vi "licenses.vi"   [LabVIEW 2019]
uses:
  <vilib>/xml/Load XML File.vi
  <vilib>/xml/Close Reference(Node).vi
  <vilib>/Utility/config.llb/Read Key (String).vi
  <vilib>/xml/NI_XML.lvlib
  <vilib>/Utility/config.llb/NI_LVConfig.lvlib
panel:
  # "This VI reads the package information from the .vipc file,\nloads the license information from the VIPM package cache,\nand stores the license text into the licenses/ directory.\n\nImportant note: This VI will only work on Windows!"
types:
  T1 = typedef "NI_LVConfig.lvlib/Config Data RefNum.ctl" = refnum<k1>
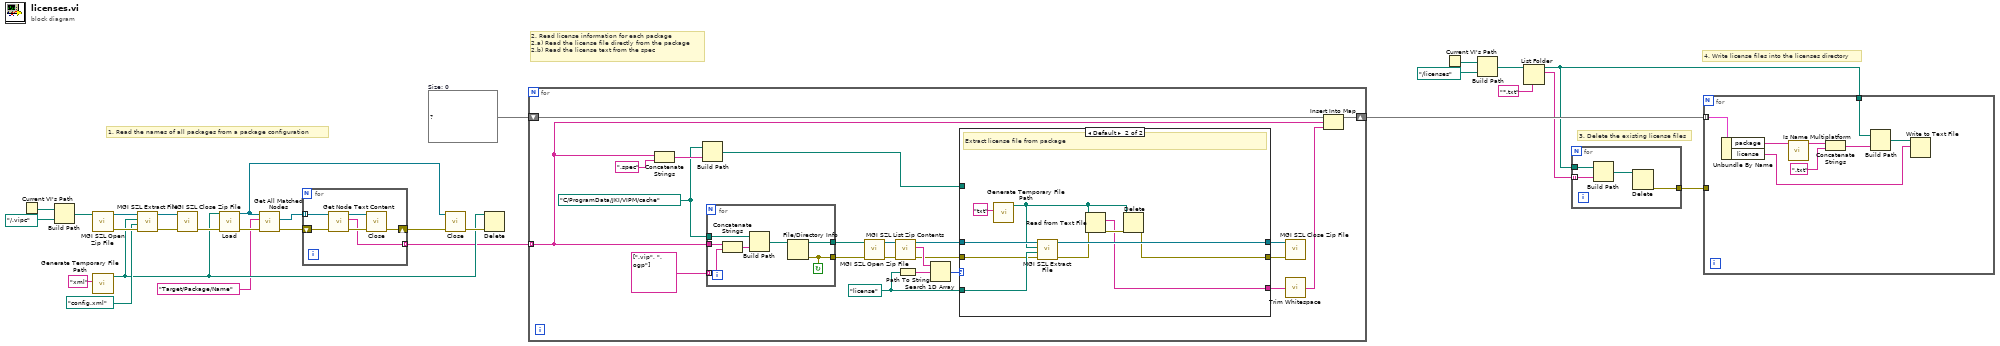
[diagram p0: block diagram]
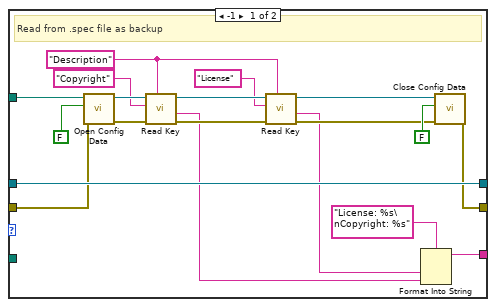
[diagram p2: hidden frame]
diagram:
  w9 = map{string, string} {}  # Size: 0
  # "3. Delete the existing license files"
  # "4. Write license files into the licenses directory"
  # "2. Read license information for each package\n2.a) Read the license file directly from the package\n2.b) Read the license text from the spec"
  # "1. Read the names of all packages from a package configuration"
  n1 = Current VI's Path() -> (path=w28:path)
  n2 = Build Path(base path=w28, name or relative path=path "../.vipc" ("Existing Zip Path")) -> (appended path=w26:path)
  n3 = call <userlib>:"MGI SZL Open Zip File.vi"("Existing Zip Path"=w26) -> ("Error Out"=w24:errorcluster, "Opened Zip File"=w25:refnum<k24>)  [unwired: 9 in]
  n4 = call <vilib>:"Generate Temporary File Path.vi"("Temporary File Extension (tmp)"="xml") -> ("Unique Temporary File Path"=w17:path)  [unwired: 9 in, 1 out]
  n5 = call <userlib>:"MGI SZL Extract File.vi"("Error In"=w24, "Entry Path In Zip"=path "config.xml", "Target Path"=w17, "Zip File"=w25) -> ("Error Out"=w20:errorcluster, "Zip File Out"=w21:refnum<k24>)  [unwired: 5 in, 1 out]
  n6 = call <userlib>:"MGI SZL Close Zip File.vi"("Error In"=w20, "Zip File"=w21) -> ("Error Out"=w19:errorcluster)  [unwired: 9 in]
  n7 = call-poly <vilib>:"Load.vi"("path to XML document"=w17, "error in (no error)"=w19) -> ("DOM document out"=w13:refnum<k20>, "error out"=w16:errorcluster)  [unwired: 11 in, 1 out]
  n8 = call <vilib>:"Get All Matched Nodes.vi"("error in (no error)"=w16, "XPath expression"="Target/Package/Name", "node in"=w13) -> ("error out"=w14:errorcluster, "node result array"=w11:refnum<k20>[])  [unwired: 6 in, 1 out]
  n9 = for {
    tunnel: w11 -> [w33] mode=indexing
    shift-right: [w30] -> w12
    shift-left: w14 -> [w34]
    tunnel: [w29] -> w10 mode=indexing
    n10 = call <vilib>:"Get Node Text Content.vi"("error in (no error)"=w34, "node in"=w33) -> ("error out"=w31:errorcluster, "node text"=w29:string, "node out"=w32:refnum<k20>)  [unwired: 7 in]
    n11 = call-poly <vilib>:"Close.vi"("error in (no error)"=w31, "node"=w32) -> ("error out"=w30:errorcluster)  [unwired: 7 in]
  }
  n12 = call-poly <vilib>:"Close.vi"("error in (no error)"=w12, "node"=w13) -> ("error out"=w18:errorcluster)  [unwired: 7 in]
  n13 = Delete(path (use dialog)=w17, error in=w18) -> ()  [unwired: 3 in, 3 out]
  n14 = for {
    tunnel: w10 -> [w38] mode=indexing
    shift-right: [w39] -> w8
    shift-left: w9 -> [w40]
    w51 = path "license" ("element")
    w42 = path "C:/ProgramData/JKI/VIPM/cache"
    n15 = Concatenate Strings(w38, ".spec" ("string")) -> (w43:string)
    n16 = Build Path(base path=w42, name or relative path=w43) -> (appended path=w41:path)
    n17 = for {
      tunnel: w38 -> [w61]
      tunnel: w42 -> [w62]
      tunnel: [w59] -> w56
      tunnel: [w58] -> w36
      tunnel: string[] [".vip", ".ogp"] -> [w57] mode=indexing
      stop <- w58 continue-if-true
      n18 = Concatenate Strings(w61, w57) -> (w63:string)
      n19 = Build Path(base path=w62, name or relative path=w63) -> (appended path=w60:path)
      n20 = File/Directory Info(path=w60) -> (path out=w59:path, error out=w58:errorcluster)  [unwired: 1 in, 5 out]
    }
    n21 = call <userlib>:"MGI SZL Open Zip File.vi"("Error In"=w36, "Existing Zip Path"=w56) -> ("Error Out"=w50:errorcluster, "Opened Zip File"=w55:refnum<k24>)  [unwired: 8 in]
    n22 = call <userlib>:"MGI SZL List Zip Contents.vi"("Error In"=w50, "Zip File"=w55) -> ("Error Out"=w49:errorcluster, "File Name[]"=w53:string[], "Zip File Out"=w54:refnum<k24>)  [unwired: 6 in, 1 out]
    n23 = Path To String(path=w51) -> (string=w52:string)
    n24 = Search 1D Array(1D array=w53, element=w52) -> (index of element=w48:i32)  [unwired: 1 in]
    n25 = case shown="Default" w48 {
      tunnel: w54 -> [w82 w91]
      tunnel: w51 -> [_ w90]
      tunnel: w49 -> [w76 w89]
      tunnel: [w82 w92] -> w47
      tunnel: [w66 w84] -> w45
      tunnel: [w75 w83] -> w46
      tunnel: w41 -> [w77 _]
      frame -1 {
        w69 = "Description" ("section")
        # "Read from .spec file as backup"
        n26 = call <vilib>:"Open Config Data.vi"("error in (no error)"=w76, "create file if necessary (T)"=FALSE, "configuration file path"=w77) -> ("error out"=w79:errorcluster, "refnum"=w80:T1)  [unwired: 6 in, 1 out]
        n27 = call-poly <vilib>:"Read Key.vi"("section"=w69, "error in (no error)"=w79, "key"="Copyright", "refnum"=w80) -> ("error out"=w70:errorcluster, "value"=w64:string, "refnum out"=w73:T1)  [unwired: 4 in, 1 out]
        n28 = call-poly <vilib>:"Read Key.vi"("section"=w69, "error in (no error)"=w70, "key"="License", "refnum"=w73) -> ("error out"=w71:errorcluster, "value"=w65:string, "refnum out"=w72:T1)  [unwired: 4 in, 1 out]
        n29 = Format Into String(format string="License: %s\nCopyright: %s", w65, w64) -> (resulting string=w66:string)  [unwired: 2 in, 1 out]
        n30 = call <vilib>:"Close Config Data.vi"("error in (no error)"=w71, "write file if changed (T)"=FALSE, "refnum"=w72) -> ("error out"=w75:errorcluster)  [unwired: 7 in, 1 out]
      }
      frame Default {
        # "Extract license file from package"
        n31 = call <vilib>:"Generate Temporary File Path.vi"("Temporary File Extension (tmp)"="txt") -> ("Unique Temporary File Path"=w85:path)  [unwired: 9 in, 1 out]
        n32 = call <userlib>:"MGI SZL Extract File.vi"("Error In"=w89, "Entry Path In Zip"=w90, "Target Path"=w85, "Zip File"=w91) -> ("Error Out"=w87:errorcluster, "Zip File Out"=w92:refnum<k24>)  [unwired: 5 in, 1 out]
        n33 = Read from Text File(file (use dialog)=w85, error in=w87) -> (text=w84:string, error out=w86:errorcluster)  [unwired: 2 in, 2 out]
        n34 = Delete(path (use dialog)=w85, error in=w86) -> (error out=w83:errorcluster)  [unwired: 3 in, 2 out]
      }
    }
    n35 = call <userlib>:"MGI SZL Close Zip File.vi"("Error In"=w46, "Zip File"=w47) -> ()  [unwired: 9 in, 1 out]
    n36 = call <vilib>:"Trim Whitespace.vi"("string"=w45) -> ("trimmed string"=w37:string)  [unwired: 1 in]
    n37 = Insert Into Map(map in=w40, key=w38, value=w37) -> (map out=w39:map{string, string})  [unwired: 2 out]
  }
  n38 = Current VI's Path() -> (path=w7:path)
  n39 = Build Path(base path=w7, name or relative path=path "../licenses" ("Existing Zip Path")) -> (appended path=w5:path)
  n40 = List Folder(path=w5, pattern="*.txt") -> (path out=w3:path, filenames=w4:string[])  [unwired: 2 in, 2 out]
  n41 = for {
    tunnel: w4 -> [w95] mode=indexing
    tunnel: w3 -> [w96]
    tunnel: [w93] -> w2
    n42 = Build Path(base path=w96, name or relative path=w95) -> (appended path=w94:path)
    n43 = Delete(path (use dialog)=w94) -> (error out=w93:errorcluster)  [unwired: 4 in, 2 out]
  }
  n44 = for {
    tunnel: w8 -> [w104] mode=indexing
    tunnel: w3 -> [w100]
    tunnel: w2 -> [_]
    n45 = Unbundle By Name(w104) -> ("package"=w103:string, "license"=w97:string)
    n46 = call <vilib>:"Is Name Multiplatform.vi"("filename"=w103) -> ("suggested filename"=w102:string)  [unwired: 6 in, 4 out]
    n47 = Concatenate Strings(w102, ".txt" ("string")) -> (w99:string)
    n48 = Build Path(base path=w100, name or relative path=w99) -> (appended path=w98:path)
    n49 = Write to Text File(file (use dialog)=w98, text=w97) -> ()  [unwired: 2 in, 3 out]
  }
